vi "LV2 Global.vi"(0 "Operation":T1, 5 "Numeric Input":dbl, 11 "Error in":errorcluster) -> (4 "Numeric Output":dbl, 15 "Error out":errorcluster)   [LabVIEW 2020]
doc: "This VI is used as a LV2 global to store and retrive data from this variable and to overcome the short comings faced from global variables"
uses:
  Typedefs/LV2 numeric.ctl
panel:
  # "LV2 Global"
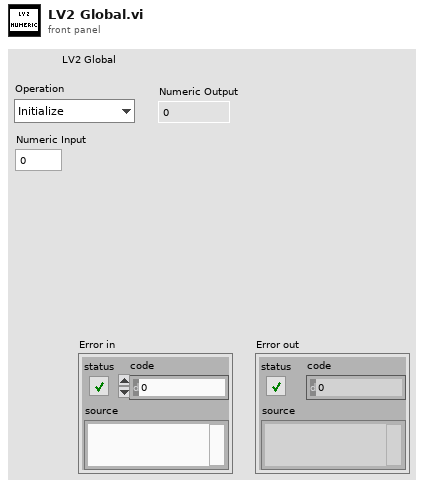
[diagram p1: front panel]
types:
  T1 = typedef "LV2 numeric.ctl" = enum16{"Initialize", "Read", "Write"}
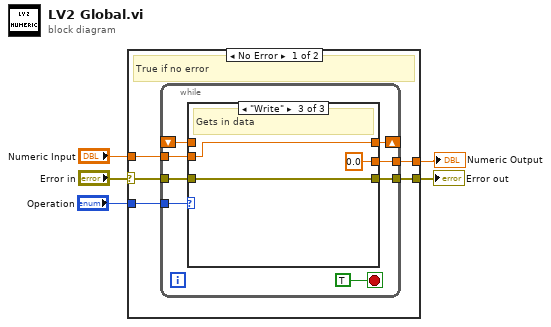
[diagram p0: block diagram]
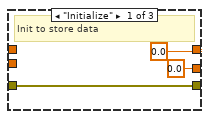
[diagram p2: hidden frame]
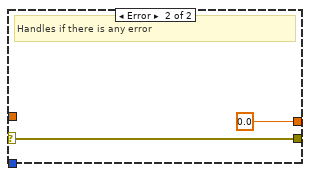
[diagram p4: hidden frame]
diagram:
  n1 = case shown="No Error" "Error in" {
    selector: "Error in" -> [w7 w28]
    tunnel: [w6 w28] -> w4
    tunnel: "Operation" -> [w10 _]
    tunnel: [w9 0.0 ("Numeric Input")] -> w2
    tunnel: "Numeric Input" -> [w8 _]
    frame No Error {
      # "True if no error"
      n2 = while {
        tunnel: w10 -> [w18]
        shift-right: [w17] -> _
        shift-left: _ -> [w16]
        tunnel: [w11] -> w9
        tunnel: w8 -> [w15]
        tunnel: w7 -> [w14]
        tunnel: [w13] -> w6
        stop <- TRUE stop-if-true
        n3 = case shown="\"Write\"" w18 {
          tunnel: [0.0 w22 w26] -> w17
          tunnel: w16 -> [_ w22 _]
          tunnel: w15 -> [_ _ w26]
          tunnel: w14 -> [w20 w23 w25]
          tunnel: [w20 w23 w25] -> w13
          tunnel: [0.0 ("Numeric Input") w22 0.0 ("Numeric Input")] -> w11
          frame "Initialize" {
            # "Init to store data"
          }
          frame "Read" {
            # "outputs data"
          }
          frame "Write" {
            # "Gets in data"
          }
        }
      }
    }
    frame Error {
      # "Handles if there is any error"
    }
  }
  "Numeric Output" <- w2
  "Error out" <- w4
